vi "LJstreamM graph processing.vi"(7 "Graph?":bool[](array[boolean]), 9 "Scan Rate":dbl=50.0 format="%.2f", 10 "Graph History (# scans)":i32 min=0, 11 "Scaled Data":dbl[][](array[numeric]) format="%.3f") -> (3 "Graph Data":cluster{dbl, dbl, dbl[][]} {"?" format="%.3f"; "?" format="%.2f"; "?" format="%.2f"})   [LabVIEW 2025]
uses:
  LJstreamM globals.vi
panel:
  out "ms":u32
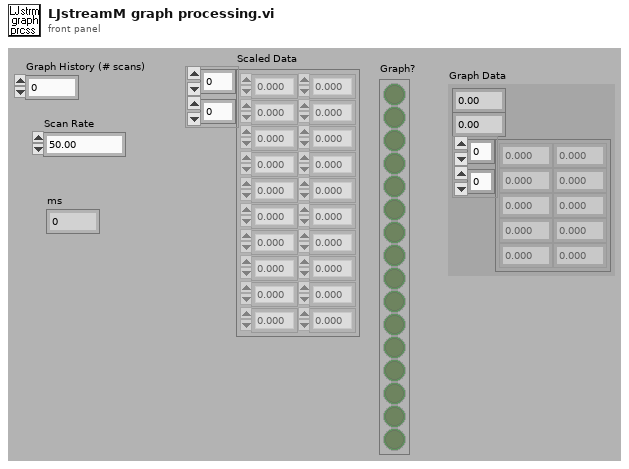
[diagram p1: front panel]
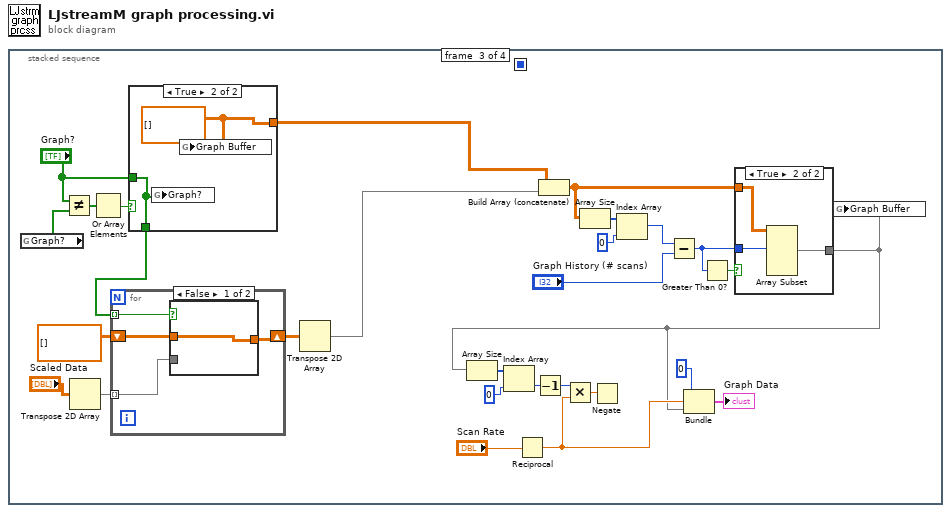
[diagram p0: block diagram]
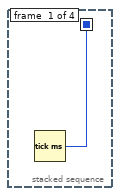
[diagram p2: hidden frame]
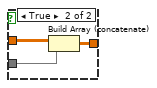
[diagram p4: hidden frame]
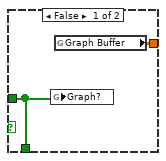
[diagram p5: hidden frame]
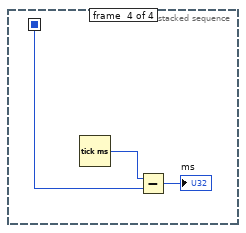
[diagram p7: hidden frame]
diagram:
  n1 = stacked-sequence {
    seq-local: [w1 _ _ _] -> [_ _ _ w47]
    frame #0 {
      n2 = Tick Count (ms)() -> (millisecond timer value=w1:u32)
    }
    frame #1 {
    }
    frame #2 {
      n3 = global read "LJstreamM globals.vi" "Graph?"() -> (w12:bool[])
      n4 = Not Equal?(x="Graph?", y=w12) -> (x != y?=w10:bool[])
      n5 = Transpose 2D Array(2D array="Scaled Data") -> (transposed array=w6:dbl[][])
      n6 = Or Array Elements(Boolean array=w10) -> (logical OR=w9:bool)
      n7 = case shown="True" w9 {
        tunnel: "Graph?" -> [w38 w41]
        tunnel: [w38 w41] -> w7
        tunnel: [w39 w40] -> w4
        frame False {
          n8 = global write "LJstreamM globals.vi" "Graph?"(w38) -> ()
          n9 = global read "LJstreamM globals.vi" "Graph Buffer"() -> (w39:dbl[][])
        }
        frame True {
          w40 = dbl[][] [] ("Graph Buffer")
          n10 = global write "LJstreamM globals.vi" "Graph?"(w41) -> ()
          n11 = global write "LJstreamM globals.vi" "Graph Buffer"(w40) -> ()
        }
      }
      n12 = for {
        tunnel: w7 -> [w33] mode=indexing
        tunnel: w6 -> [w32] mode=indexing
        shift-right: [w31] -> w3
        shift-left: dbl[][] [] -> [w30]
        n13 = case shown="False" w33 {
          tunnel: w32 -> [_ w37]
          tunnel: [w34 w36] -> w31
          tunnel: w30 -> [w34 w35]
          frame False {
          }
          frame True {
            n14 = Build Array (concatenate)(w35, w37) -> (w36:dbl[][])
          }
        }
      }
      n15 = Transpose 2D Array(2D array=w3) -> (transposed array=w2:dbl[][])
      n16 = Reciprocal(x="Scan Rate") -> (1/x=w16:dbl)
      n17 = Build Array (concatenate)(w4, w2) -> (w23:dbl[][])
      n18 = Array Size(array=w23) -> (size(s)=w29:i32[])
      n19 = Index Array(array=w29, index=0 ("Index")) -> (element=w27:i32)
      n20 = Subtract(x=w27, y="Graph History (# scans)") -> (x-y=w24:i32)
      n21 = Greater Than 0?(x=w24) -> (x > 0?=w25:bool)
      n22 = case shown="True" w25 {
        tunnel: w24 -> [_ w45]
        tunnel: w23 -> [w42 w44]
        tunnel: [w42 w43] -> w13
        frame False {
        }
        frame True {
          n23 = Array Subset(array=w44, index (row)=w45) -> (w43:dbl[][])  [unwired: 3 in]
        }
      }
      n24 = Array Size(array=w13) -> (size(s)=w20:i32[])
      n25 = Index Array(array=w20, index=0 ("Index")) -> (element=w19:i32)
      n26 = Decrement(x=w19) -> (x-1=w18:i32)
      n27 = Multiply(x=w18, y=w16) -> (x*y=w17:dbl)
      n28 = Negate(x=w17) -> ()  [unwired: 1 out]
      n29 = Bundle(0, w16, w13) -> (→"Graph Data":cluster{i32, dbl, dbl[][]})  [unwired: 1 in]
      n30 = global write "LJstreamM globals.vi" "Graph Buffer"(w13) -> ()
    }
    frame #3 {
      n31 = Tick Count (ms)() -> (millisecond timer value=w48:u32)
      n32 = Subtract(x=w48, y=w47) -> (x-y=→"ms":u32)
    }
  }
